vi "Autonomous_v204.vi"() -> ()   [LabVIEW 2017]
doc: "This VI starts when autonomous period begins, and will automatically be terminated when it ends. You can carry out timed or sensor driven operations directly to I/O or to subsystems without needing to return to the caller."
uses:
  <vilib>/Rock Robotics/Network Tables/NT Read String.vi
panel:
  out "RightArmMotorCmd 2":dbl(graph)
  out "Lift Min Limit  2":bool
  out "Lift Max Limit 2":bool
  out "LiftMotorCmd 2":dbl(graph)
  out "Left Arm Max Limit 2":bool
  out "Right Arm Max Limit 2":bool
  out "Right Arm Min Limit 2":bool
  out "Left Arm Min Limit 2":bool
  out "LeftArmMotorCmd 2":dbl(graph)
  out "Arm Lift Min Limit  2":bool
  out "Arm Lift Max Limit  2":bool
  out "ArmLiftMotorCmd 2":dbl(graph)
  out "Waveform Chart 6":dbl(graph)
  out "Waveform Chart 15":dbl(graph)
  out "Waveform Chart 10":dbl(graph)
  out "millisecond timer value 3":u32
  out "String 2":string
  out "Waveform Chart 45":i32(graph)
  out "Waveform Chart 44":i32(graph)
  out "Waveform Chart 43":i32(graph)
  out "Waveform Chart 42":i32(graph)
  out "Waveform Chart 14":i32(graph)
  out "Waveform Chart 12":i32(graph)
  out "Waveform Chart 41":i32(graph)
  out "Waveform Chart 40":i32(graph)
  out "Waveform Chart 39":i32(graph)
  out "Waveform Chart 38":i32(graph)
  out "Waveform Chart 37":i32(graph)
  out "Waveform Chart 36":i32(graph)
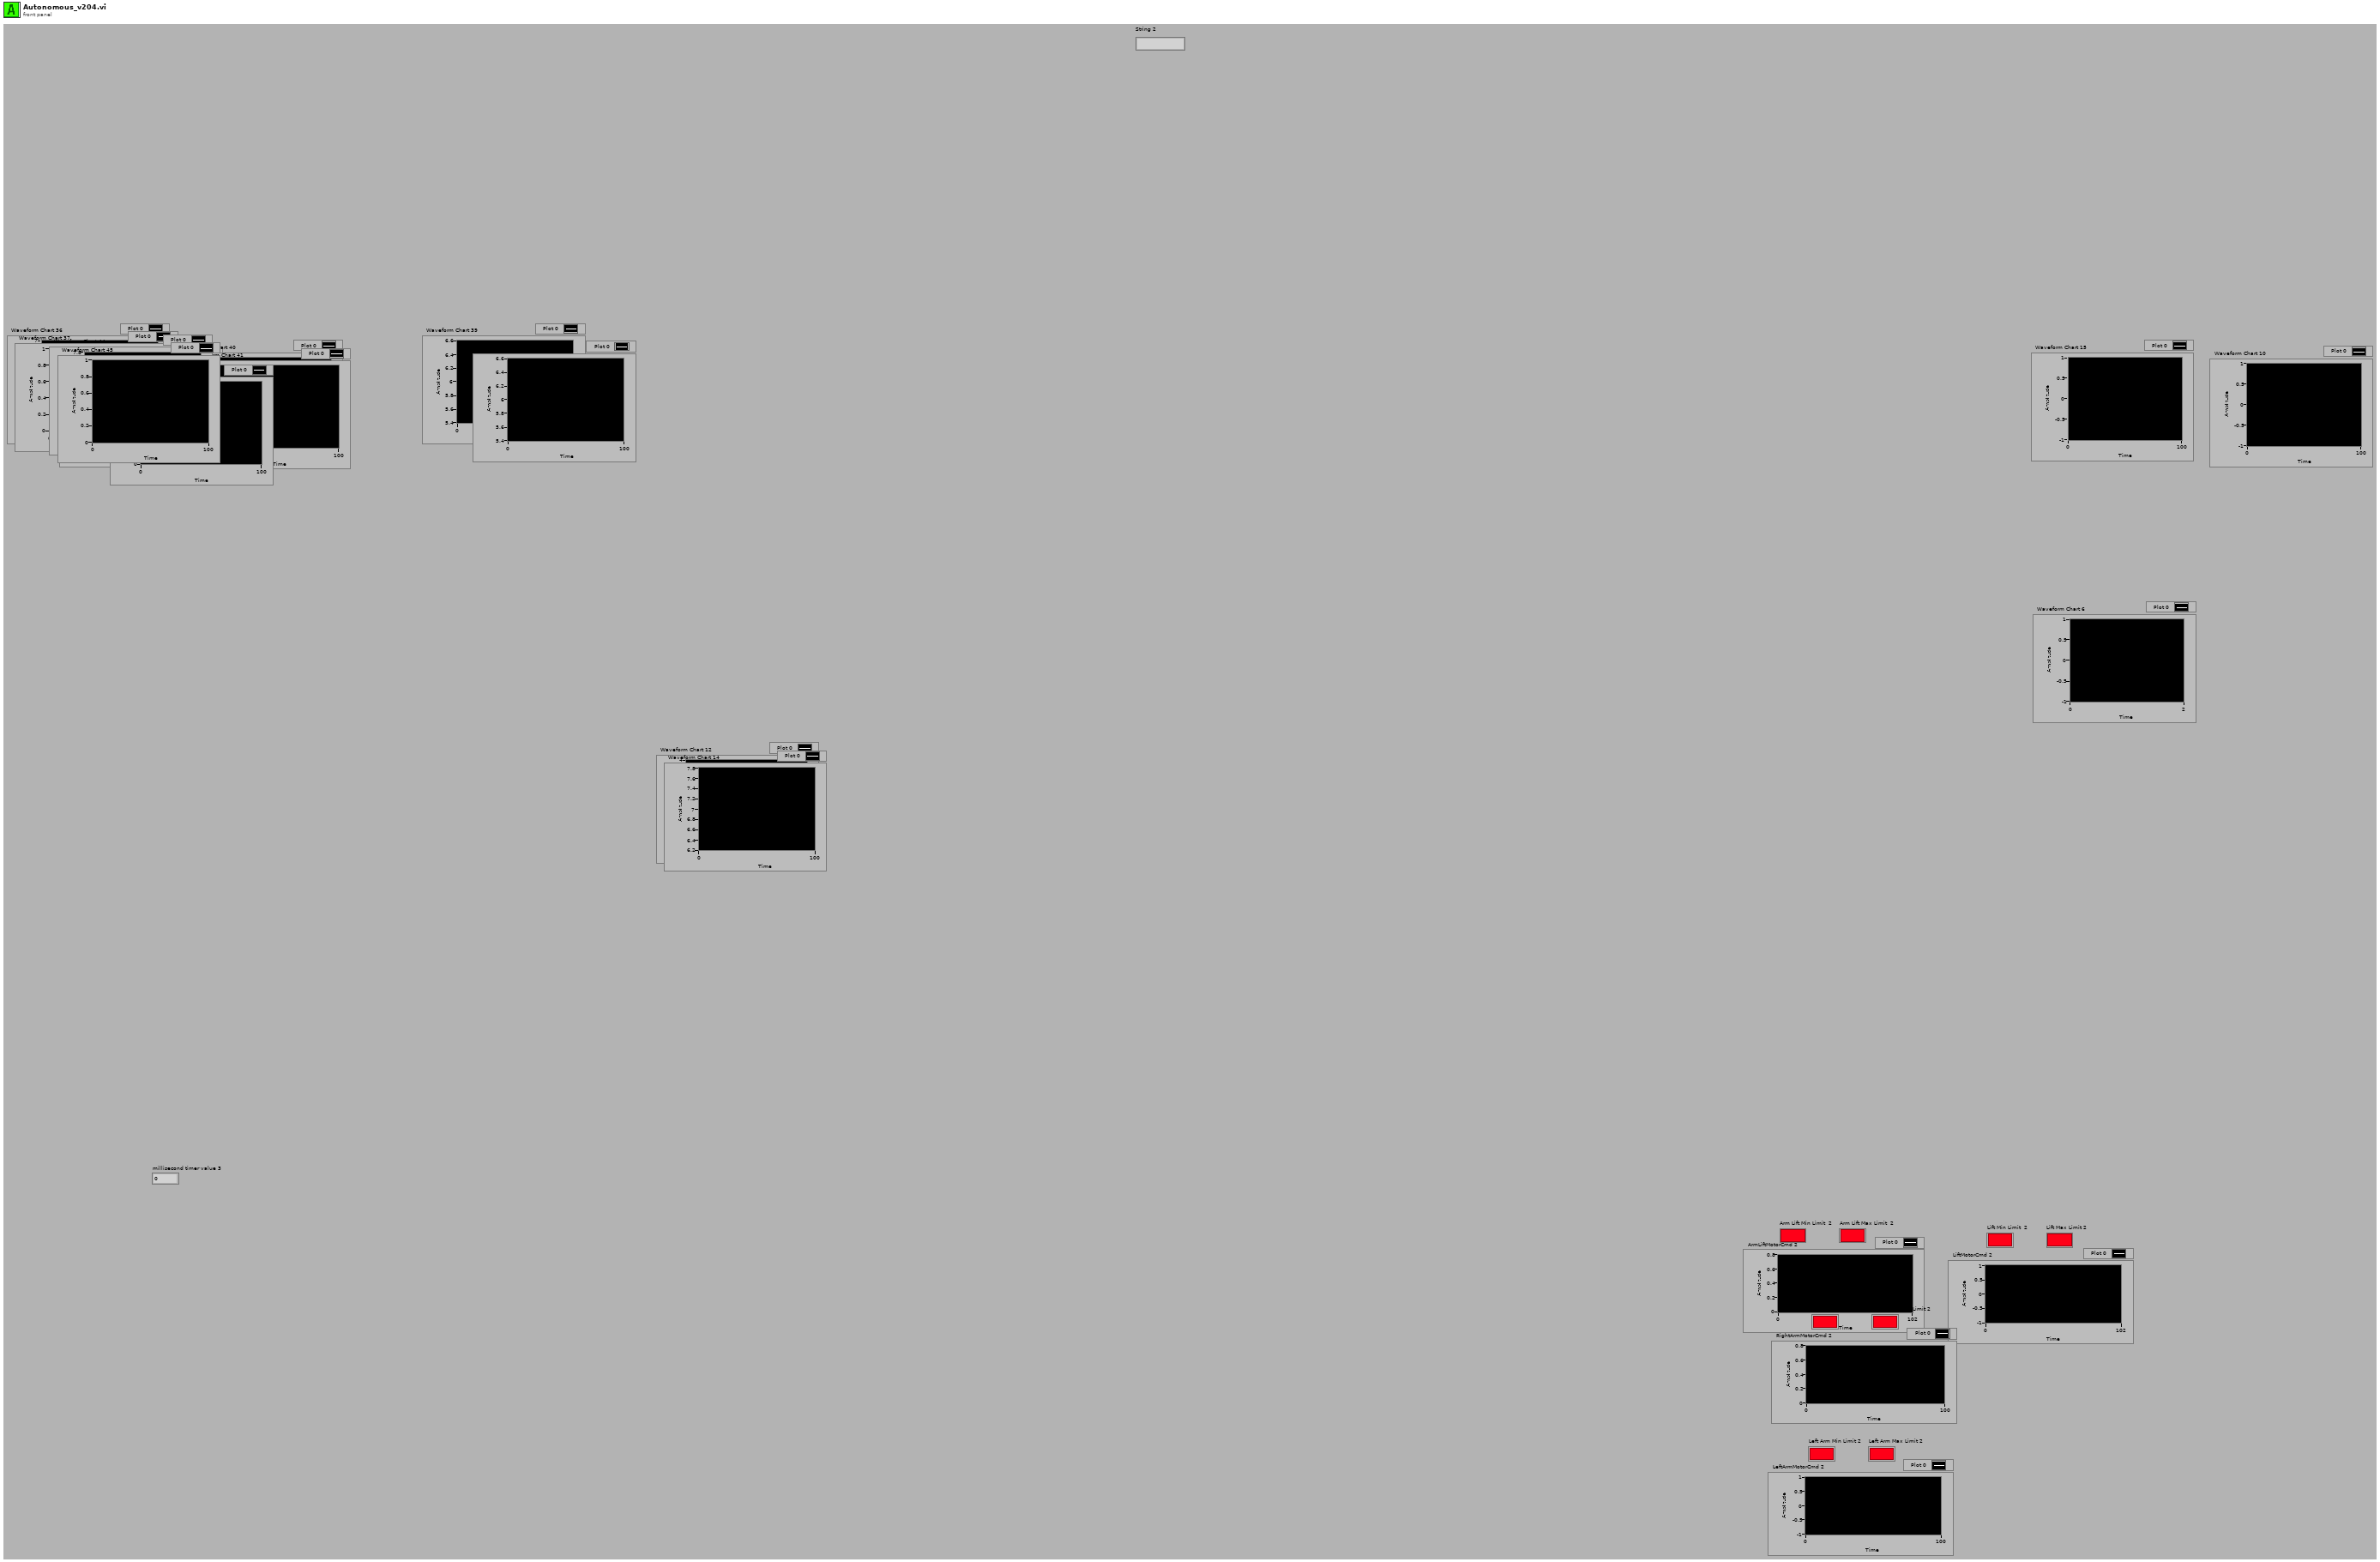
[diagram p1: front panel]
types:
  T1 = cluster{"X_axis":dbl, "Y_axis":dbl, "RotationTarget":dbl, "ArmLift":dbl, "Hands":dbl, "Lift":dbl, "Arms":dbl}
  T2 = enum16{"initialize", "read", "write", "write all"}
  T3 = typedef "DioDisplayALB.ctl" = cluster{"DIO 0-LiftMinLimitSwitch":bool, "DIO 1-LiftMaxLimitSwitch":bool, "DIO 2-LiftArmMinLimitSwitch":bool, "DIO 3-LiftArmMaxLimitSwitch":bool, "DIO 4-RightArmMaxLimitSwitch":bool, "DIO 5-RightArmMinLimitSwitch":bool, "DIO 6-LeftArmMaxLimitSwitch":bool, "DIO 7-LeftArmMinLimitSwitch":bool, "DIO 8":bool, "DIO 9":bool}
  T4 = typedef "WPI_MotorControlDeviceRef.ctl" = cluster{"DeviceStatus":errorcluster, "Type":T5, "PWM":cluster{"PWM Channel":T6, "DeadBand":T7}, "CAN":cluster{"Device Number":u8, "SetOutput VI Ref":variant, "GetOutput VI Ref":variant, "Enable VI Ref":variant, "Disable VI Ref":variant, "Data":variant}, "Invert":bool, "DIO PWM":cluster{"PWM \"Enable\" Channel":T6, "DIOChannel":T8, "PWM Rate":dbl}}
  T5 = typedef "WPI_MotorControlType.ctl" = enum16{"PWM", "CAN", "DIO PWM"}
  T6 = typedef "FPGA_DIOPWMChannel.ctl" = enum8{"PWM 0", "PWM 1", "PWM 2", "PWM 3", "PWM 4", "PWM 5", "PWM 6", "PWM 7", "PWM 8", "PWM 9", "PWM MXP 0", "PWM MXP 1", "PWM MXP 2", "PWM MXP 3", "PWM MXP 4", "PWM MXP 5", "PWM MXP 6", "PWM MXP 7", "PWM MXP 8", "PWM MXP 9", "Invalid"}
  T7 = typedef "WPI_PWMDeadband.ctl" = cluster{"Name":string, "maxPositivePwm":i32, "minPositivePwm":i32, "centerPwm":i32, "maxNegativePwm":i32, "minNegativePwm":i32, "angularRange":u16}
  T8 = typedef "FPGA_DIOChannel.ctl" = enum8{"DIO 0", "DIO 1", "DIO 2", "DIO 3", "DIO 4", "DIO 5", "DIO 6", "DIO 7", "DIO 8", "DIO 9", "DIO MXP 0", "DIO MXP 1", "DIO MXP 2", "DIO MXP 3", "DIO MXP 4", "DIO MXP 5", "DIO MXP 6", "DIO MXP 7", "DIO MXP 8", "DIO MXP 9", "DIO MXP 10", "DIO MXP 11", "DIO MXP 12", "DIO MXP 13", "DIO MXP 14", "DIO MXP 15", "SPI Port CS1", "SPI Port CS2", "SPI Port CS3", "SPI Port MISO", "SPI Port MOSI", "Invalid"}
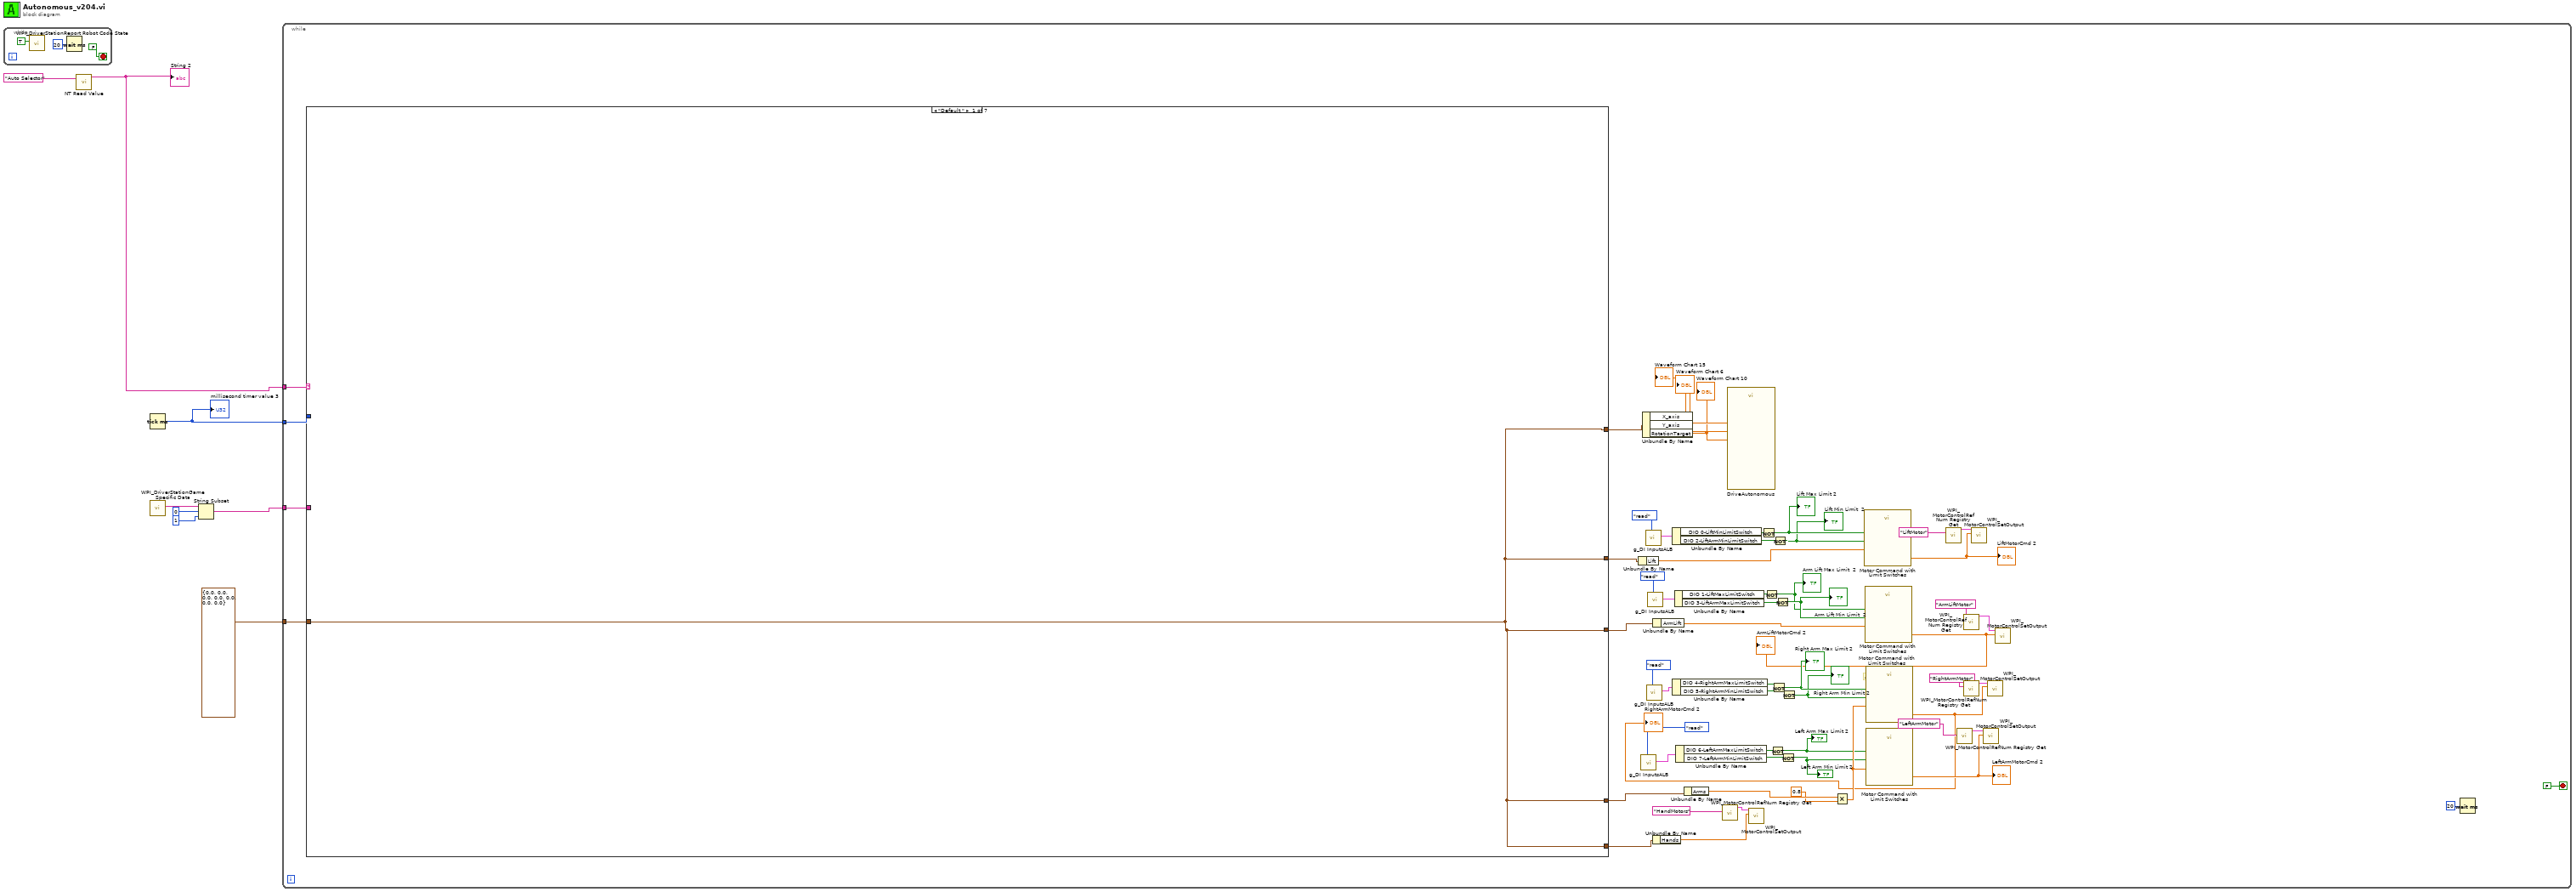
[diagram p0: block diagram]
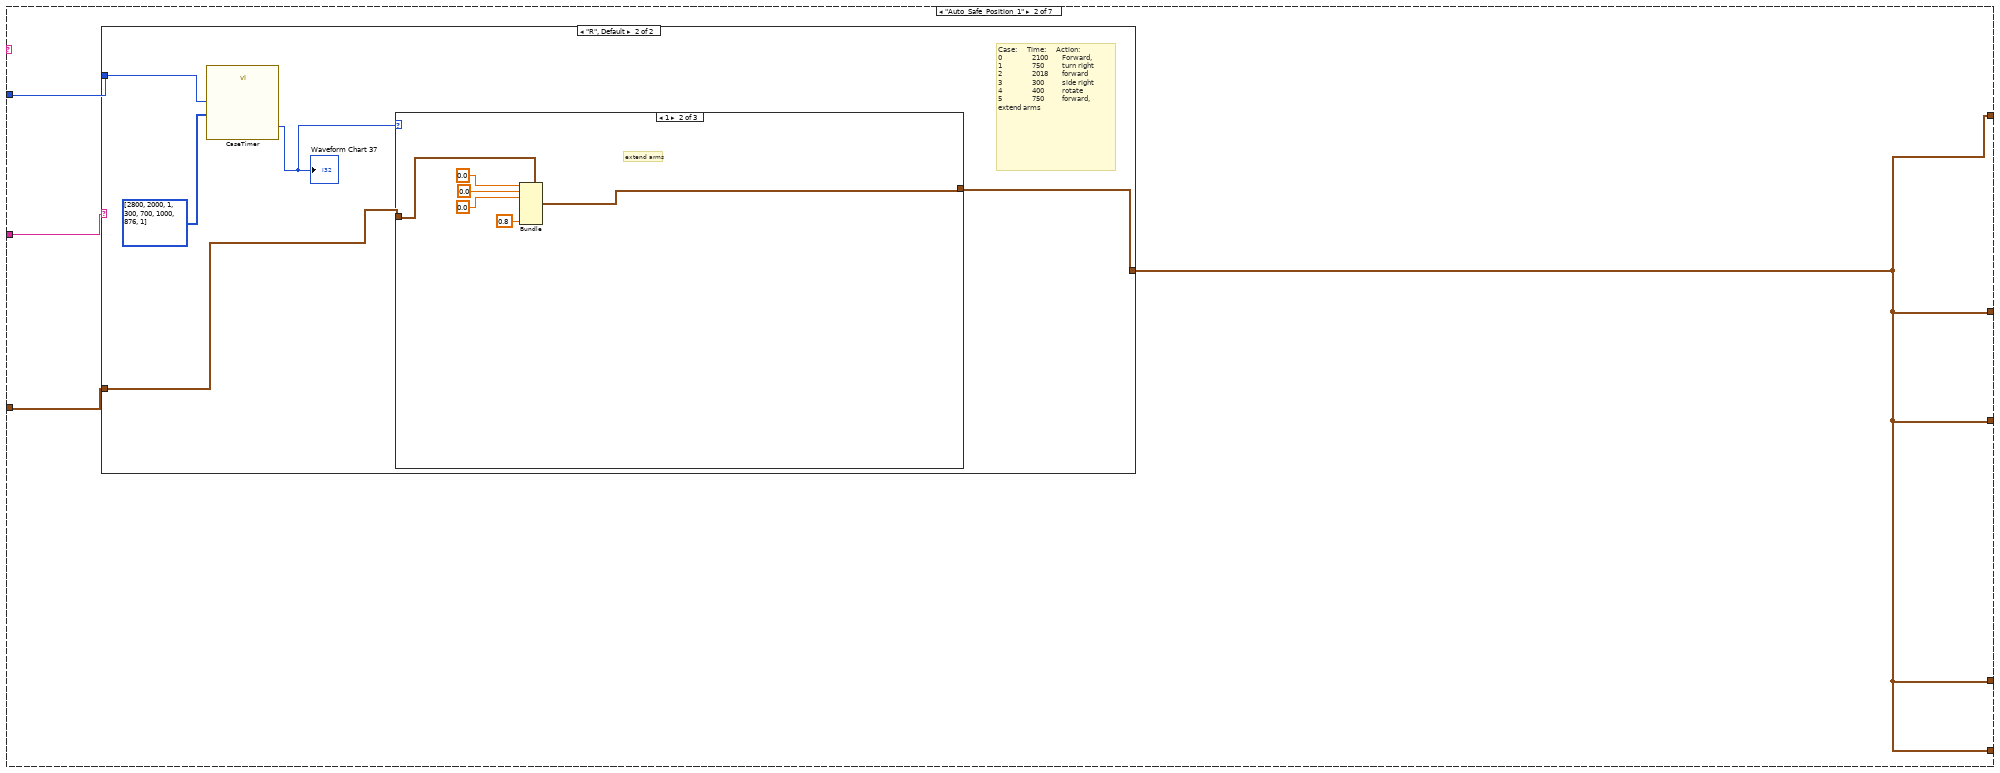
[diagram p2: hidden frame]
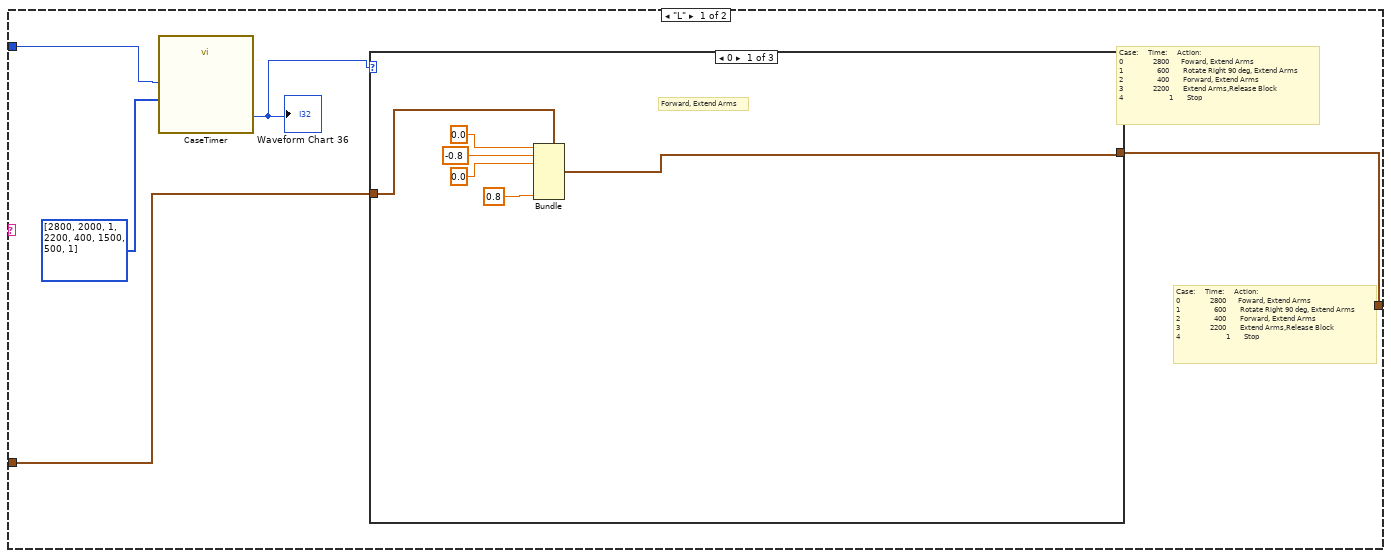
[diagram p3: hidden frame]
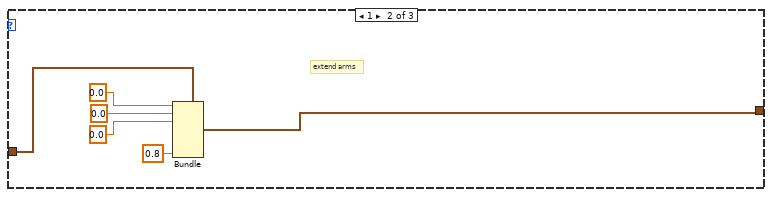
[diagram p4: hidden frame]
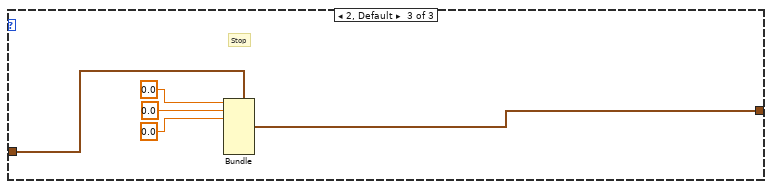
[diagram p5: hidden frame]
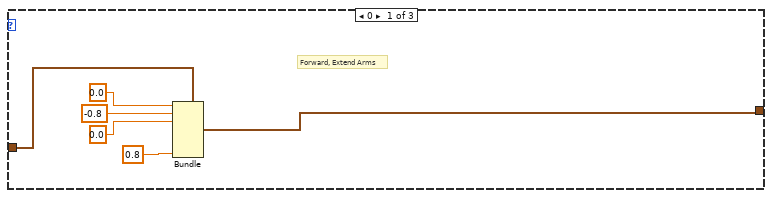
[diagram p6: hidden frame]
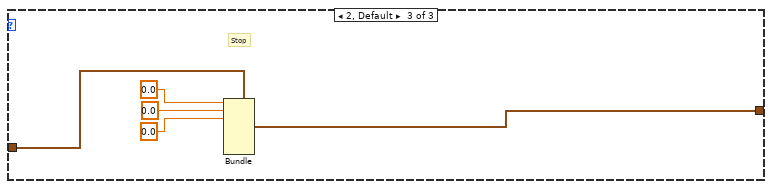
[diagram p7: hidden frame]
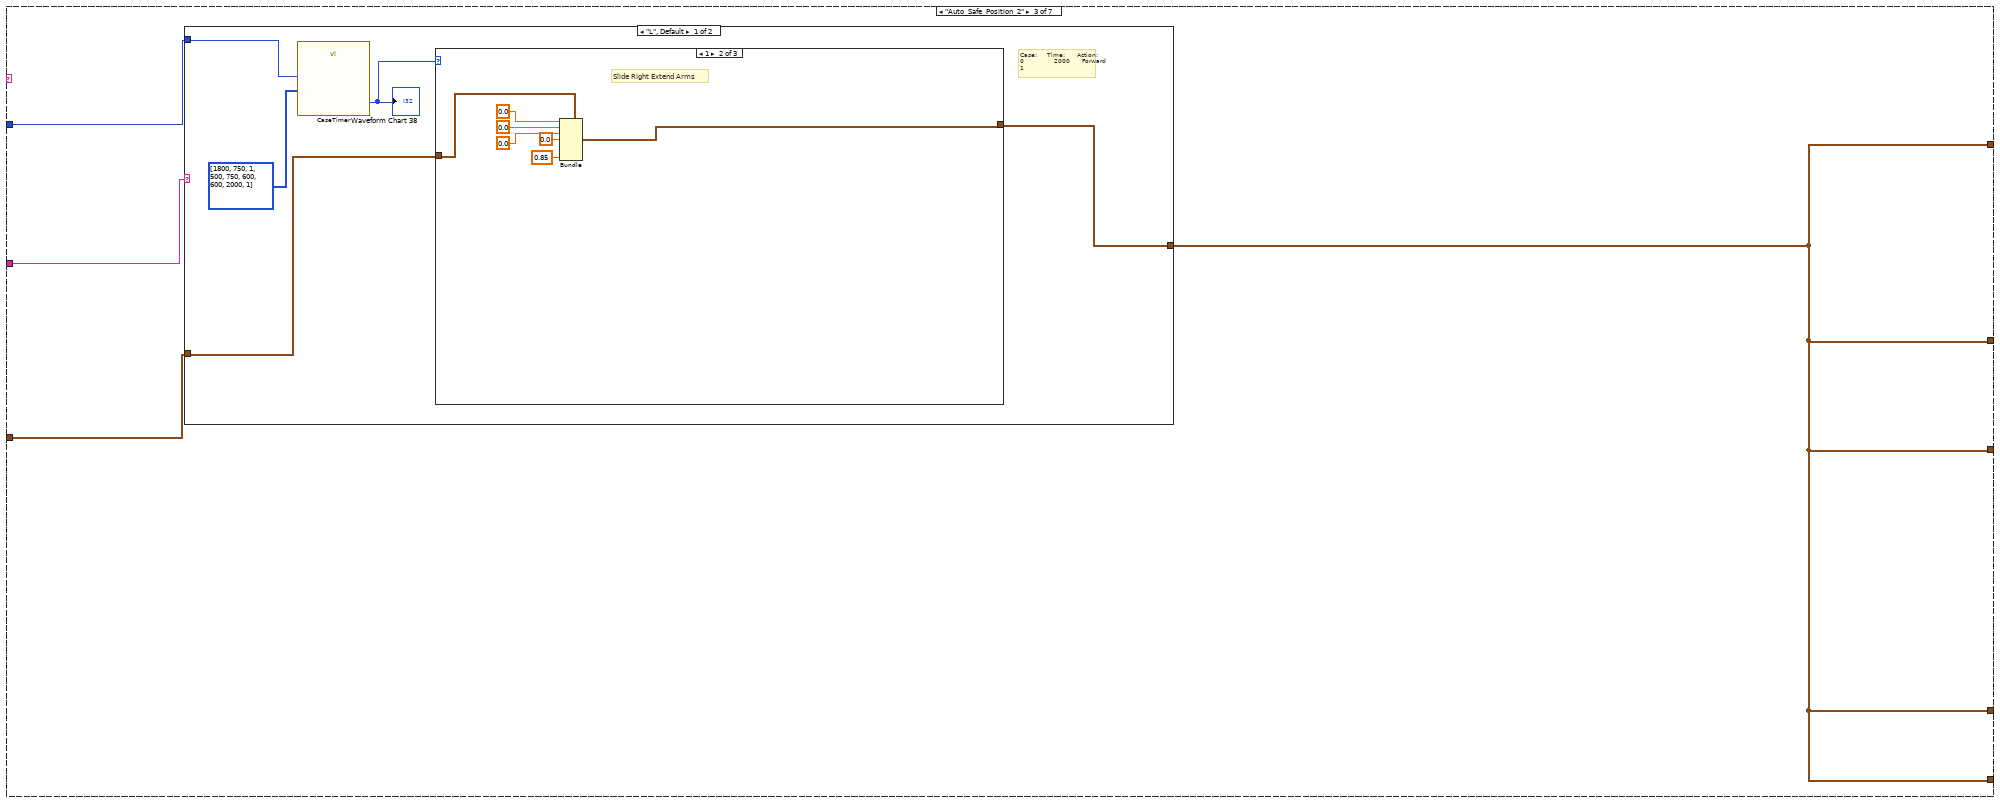
[diagram p8: hidden frame]
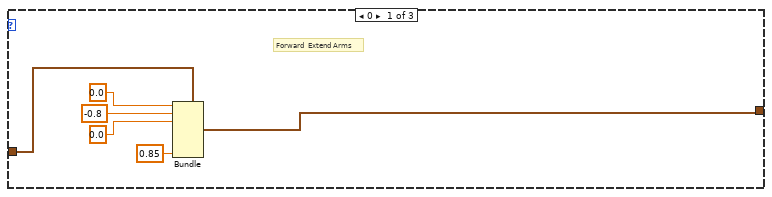
[diagram p9: hidden frame]
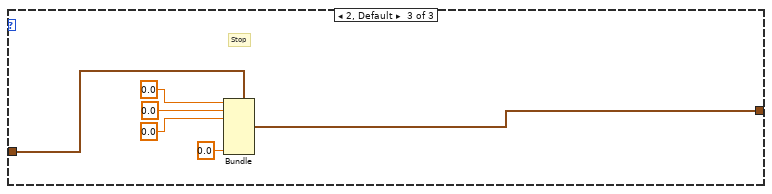
[diagram p10: hidden frame]
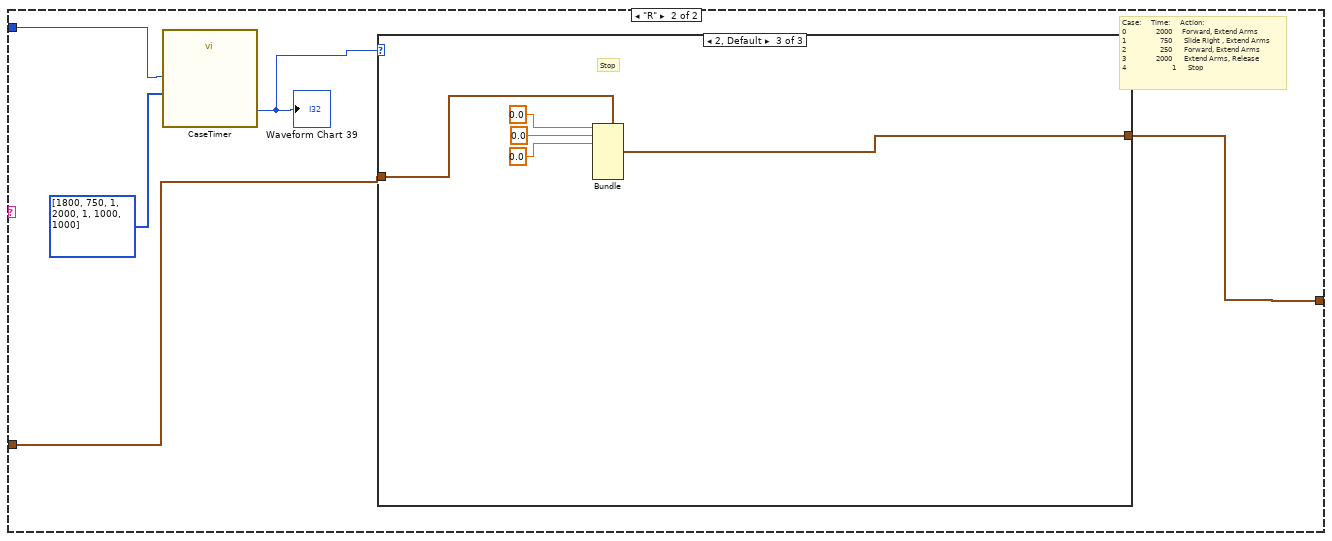
[diagram p11: hidden frame]
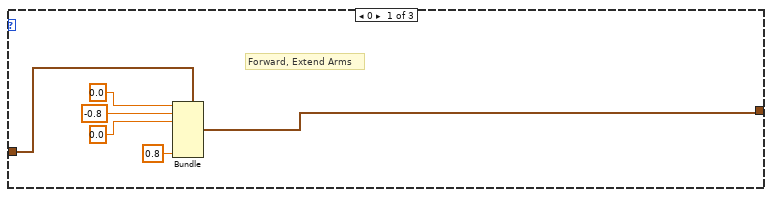
[diagram p12: hidden frame]
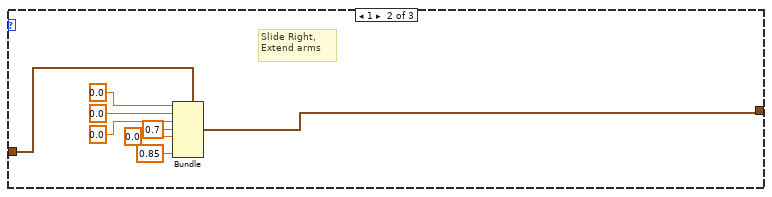
[diagram p13: hidden frame]
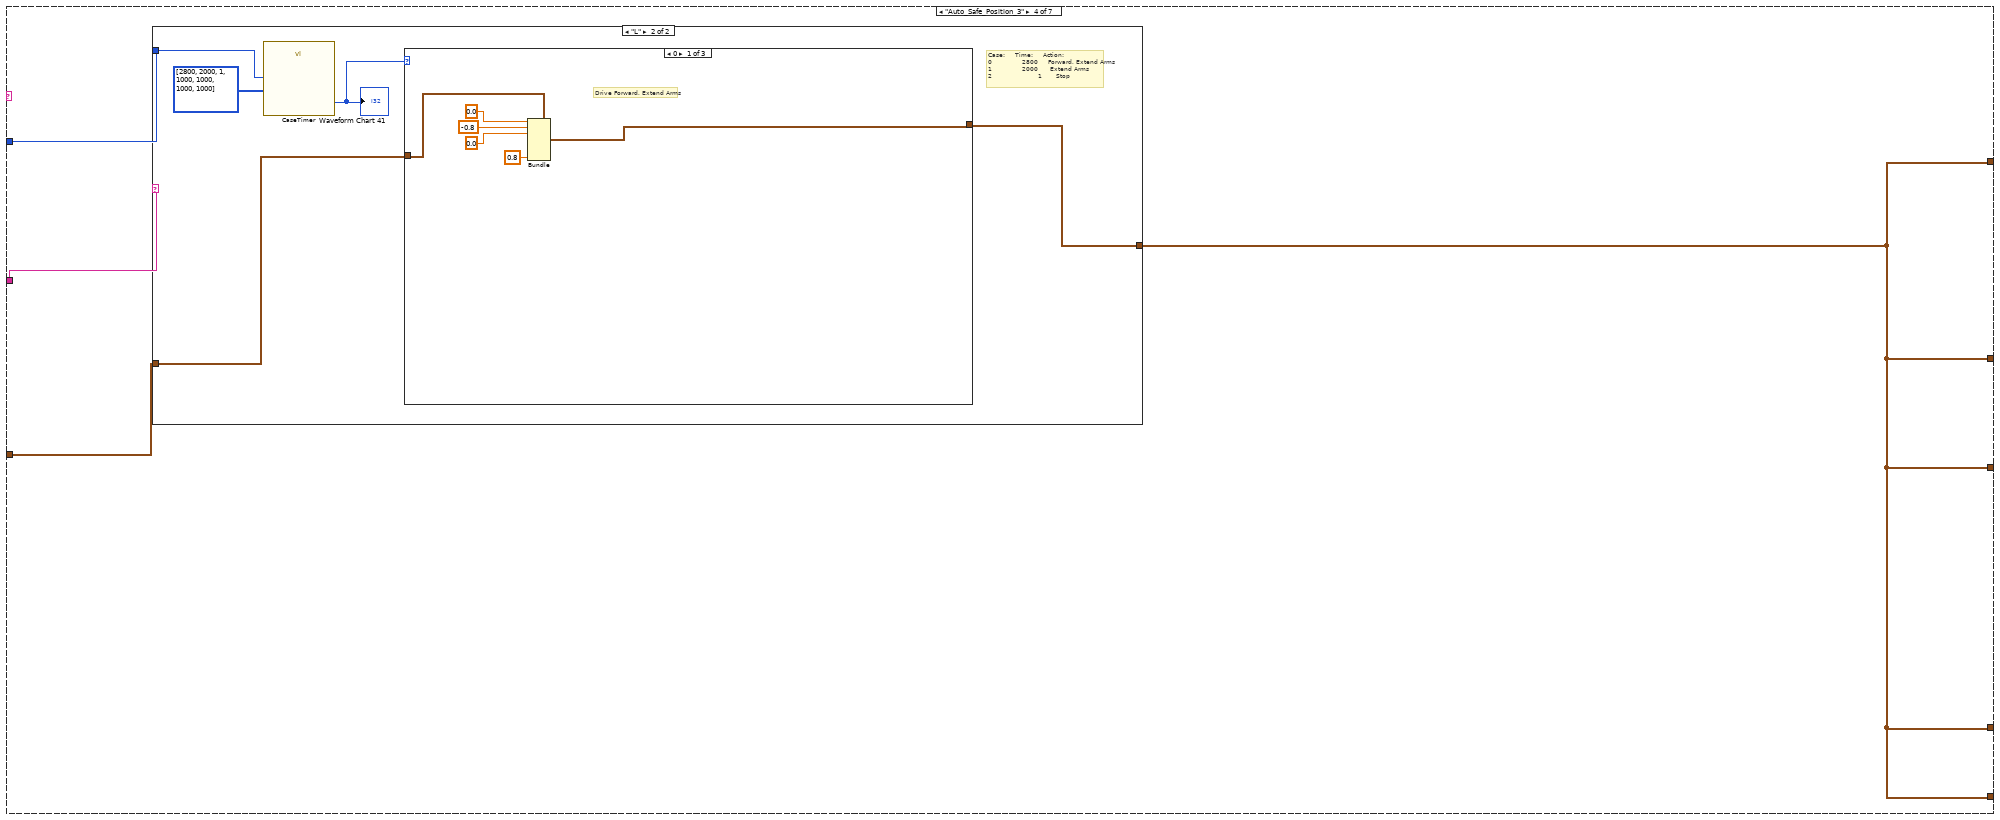
[diagram p14: hidden frame]
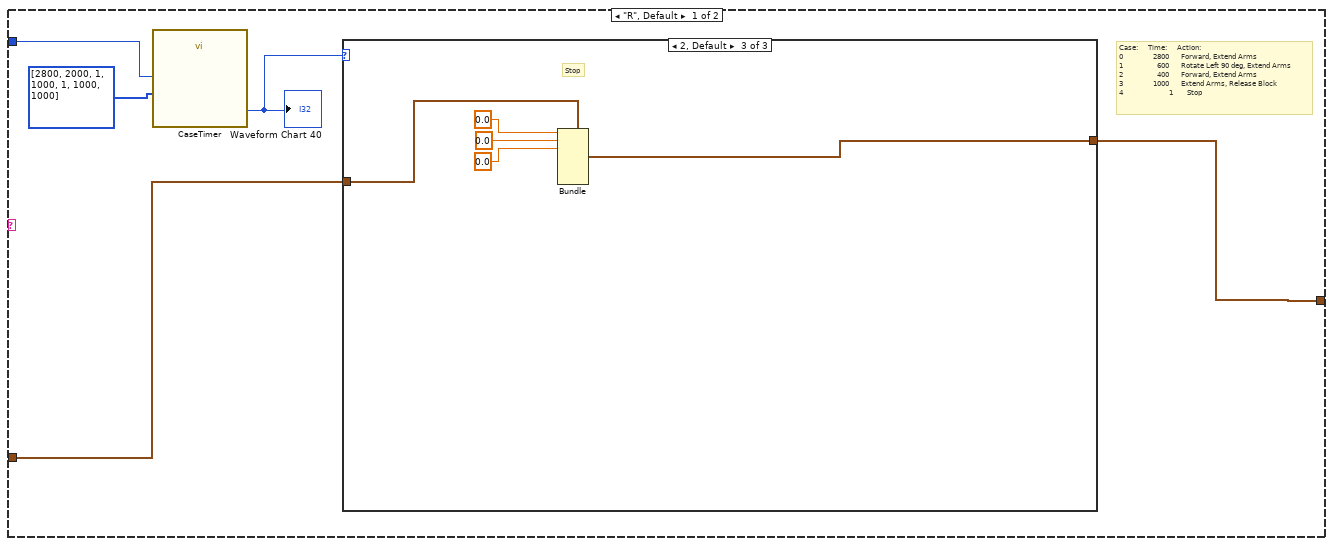
[diagram p15: hidden frame]
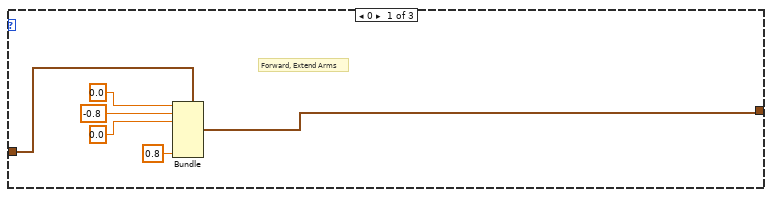
[diagram p16: hidden frame]
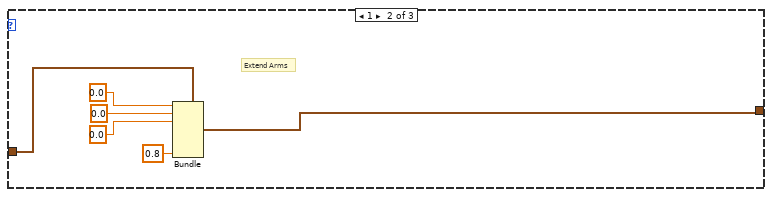
[diagram p17: hidden frame]
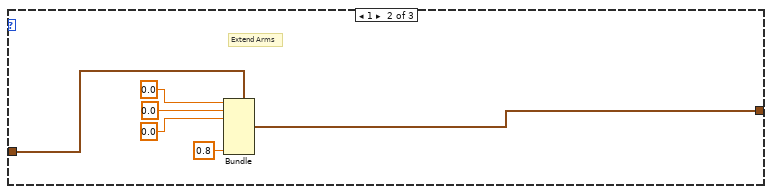
[diagram p18: hidden frame]
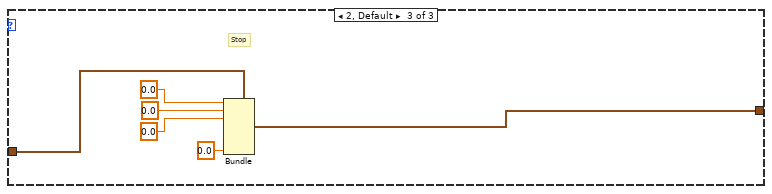
[diagram p19: hidden frame]
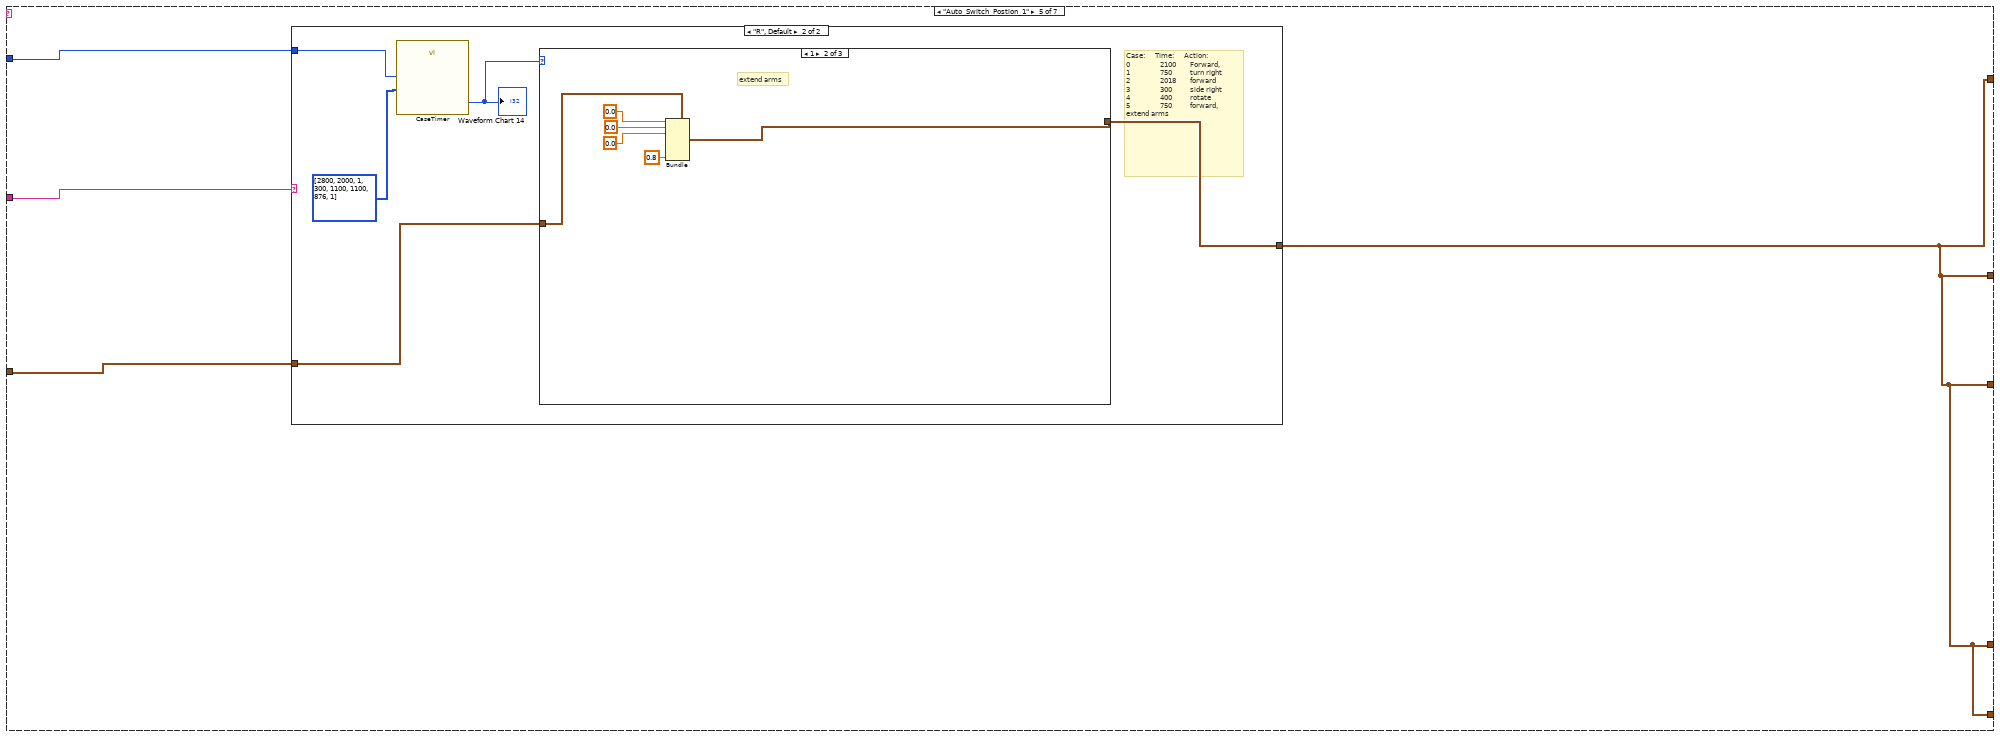
[diagram p20: hidden frame]
diagram:
  n1 = while {
    stop <- FALSE stop-if-true
    n2 = call <vilib>:"WPI_DriverStationReport Robot Code State.vi"("Autonomous"=TRUE) -> ()  [unwired: 10 in, 1 out]
    n3 = Wait (ms)(milliseconds to wait=u32 20) -> ()  [unwired: 1 out]
  }
  n4 = call-poly <vilib>:"NT Read Value.vi"("Name"="Auto Selector") -> ("String"=w1:string)  [unwired: 9 in, 1 out]
  "String 2" <- w1
  n5 = call <vilib>:"WPI_DriverStationGame Specific Data.vi"() -> ("Game Specific Data"=w7:string)  [unwired: 11 in]
  n6 = Tick Count (ms)() -> (millisecond timer value=w2:u32)
  "millisecond timer value 3" <- w2
  n7 = String Subset(string=w7, offset (0)=0, length (rest)=1 ("length (rest)")) -> (substring=w3:string)
  n8 = while {
    tunnel: T1 {"X_axis"=0.0, "Y_axis"=0.0, "RotationTarget"=0.0, "ArmLift"=0.0, "Hands"=0.0, "Lift"=0.0, "Arms"=0.0} ("Cluster") -> [w68]
    tunnel: w3 -> [w67]
    tunnel: w2 -> [w66]
    tunnel: w1 -> [w65]
    stop <- FALSE stop-if-true
    # "Arms"
    n9 = case shown="\"Default \"" w65 {
      tunnel: w66 -> [_ w73 w119 w174 w222 w302 w359]
      tunnel: w68 -> [w70 w72 w121 w172 w221 w300 w361]
      tunnel: w67 -> [_ w74 w122 w173 w223 w301 w362]
      tunnel: [w70 w71 w120 w171 w220 w299 w360] -> w15
      tunnel: [w70 w71 w120 w171 w220 w299 w360] -> w17
      tunnel: [w70 w71 w120 w171 w220 w299 w360] -> w16
      tunnel: [w70 w71 w120 w171 w220 w299 w360] -> w14
      tunnel: [w70 w71 w120 w171 w220 w299 w360] -> w18
      frame "Default " {
      }
      frame "Auto_Safe_Position_1" {
        n10 = case shown="\"R\", Default" w74 {
          tunnel: w72 -> [w77 w99]
          tunnel: [w75 w97] -> w71
          tunnel: w73 -> [w79 w101]
          frame "L" {
            # "Case:     Time:     Action:\n0               2800      Foward, Extend Arms\n1                 600       Rotate Right 90 deg, Extend Arms\n2                 400       Forward, Extend Arms\n3               2200       Extend Arms,Release Block\n4                       1       Stop"
            # "Case:     Time:     Action:\n0               2800      Foward, Extend Arms\n1                 600       Rotate Right 90 deg, Extend Arms\n2                 400       Forward, Extend Arms\n3               2200       Extend Arms,Release Block\n4                       1       Stop"
            n11 = call "CaseTimer.vi"("CaseTime"=u32[] [2800, 2000, 1, 2200, 400, 1500, 500, 1] ("y"), "ElapsedTime"=w79) -> ("CaseNumber"=w76:i32)  [unwired: 9 in]
            "Waveform Chart 36" <- w76
            n12 = case shown="0" w76 {
              tunnel: [w82 w88 w93] -> w75
              tunnel: w77 -> [w80 w86 w92]
              frame 0 {
                # "Forward, Extend Arms"
                n13 = Bundle(cluster=w80, "X_axis"=0.0, "Y_axis"=-0.8, "RotationTarget"=0.0, "Arms"=0.8) -> (w82:T1)  [unwired: 3 in]
              }
              frame 1 {
                # "extend arms"
                n14 = Bundle(cluster=w86, "X_axis"=0.0, "Y_axis"=0.0, "RotationTarget"=0.0, "Arms"=0.8) -> (w88:T1)  [unwired: 3 in]
              }
              frame 2, Default {
                # "Stop"
                n15 = Bundle(cluster=w92, "X_axis"=0.0, "Y_axis"=0.0, "RotationTarget"=0.0) -> (w93:T1)  [unwired: 4 in]
              }
            }
          }
          frame "R", Default {
            # "Case:     Time:     Action:\n0               2100       Forward, \n1               750         turn right\n2               2018       forward\n3               300         side right\n4               400         rotate\n5               750         forward, extend arms"
            n16 = call "CaseTimer.vi"("CaseTime"=u32[] [2800, 2000, 1, 300, 700, 1000, 876, 1] ("y"), "ElapsedTime"=w101) -> ("CaseNumber"=w98:i32)  [unwired: 9 in]
            "Waveform Chart 37" <- w98
            n17 = case shown="1" w98 {
              tunnel: [w104 w110 w115] -> w97
              tunnel: w99 -> [w102 w108 w114]
              frame 0 {
                # "Forward, Extend Arms"
                n18 = Bundle(cluster=w102, "X_axis"=0.0, "Y_axis"=-0.8, "RotationTarget"=0.0, "Arms"=0.8) -> (w104:T1)  [unwired: 3 in]
              }
              frame 1 {
                # "extend arms"
                n19 = Bundle(cluster=w108, "X_axis"=0.0, "Y_axis"=0.0, "RotationTarget"=0.0, "Arms"=0.8) -> (w110:T1)  [unwired: 3 in]
              }
              frame 2, Default {
                # "Stop"
                n20 = Bundle(cluster=w114, "X_axis"=0.0, "Y_axis"=0.0, "RotationTarget"=0.0) -> (w115:T1)  [unwired: 4 in]
              }
            }
          }
        }
      }
      frame "Auto_Safe_Position_2" {
        n21 = case shown="\"L\", Default" w122 {
          tunnel: w121 -> [w127 w149]
          tunnel: [w126 w147] -> w120
          tunnel: w119 -> [w124 w151]
          frame "L", Default {
            # "Case:     Time:      Action:\n0               2000      Forward\n1"
            n22 = call "CaseTimer.vi"("CaseTime"=u32[] [1800, 750, 1, 500, 750, 600, 600, 2000, 1] ("y"), "ElapsedTime"=w124) -> ("CaseNumber"=w125:i32)  [unwired: 9 in]
            "Waveform Chart 38" <- w125
            n23 = case shown="1" w125 {
              tunnel: w127 -> [w130 w137 w146]
              tunnel: [w129 w136 w142] -> w126
              frame 0 {
                # "Forward  Extend Arms"
                n24 = Bundle(cluster=w130, "X_axis"=0.0, "Y_axis"=-0.8, "RotationTarget"=0.0, "Arms"=0.85) -> (w129:T1)  [unwired: 3 in]
              }
              frame 1 {
                # "Slide RIght Extend Arms"
                n25 = Bundle(cluster=w137, "X_axis"=0.0, "Y_axis"=0.0, "RotationTarget"=0.0, "ArmLift"=0.0, "Arms"=0.85) -> (w136:T1)  [unwired: 2 in]
              }
              frame 2, Default {
                # "Stop"
                n26 = Bundle(cluster=w146, "X_axis"=0.0, "Y_axis"=0.0, "RotationTarget"=0.0, "Arms"=0.0) -> (w142:T1)  [unwired: 3 in]
              }
            }
          }
          frame "R" {
            # "Case:     Time:     Action:\n0               2000     Forward, Extend Arms\n1                 750      Slide Right , Extend Arms\n2                 250      Forward, Extend Arms\n3               2000      Extend Arms, Release\n4                       1      Stop"
            n27 = call "CaseTimer.vi"("CaseTime"=u32[] [1800, 750, 1, 2000, 1, 1000, 1000] ("y"), "ElapsedTime"=w151) -> ("CaseNumber"=w148:i32)  [unwired: 9 in]
            "Waveform Chart 39" <- w148
            n28 = case shown="2, Default" w148 {
              tunnel: w149 -> [w154 w162 w170]
              tunnel: [w153 w161 w166] -> w147
              frame 0 {
                # "Forward, Extend Arms"
                n29 = Bundle(cluster=w154, "X_axis"=0.0, "Y_axis"=-0.8, "RotationTarget"=0.0, "Arms"=0.8) -> (w153:T1)  [unwired: 3 in]
              }
              frame 1 {
                # "Slide Right, Extend arms"
                n30 = Bundle(cluster=w162, "X_axis"=0.0, "Y_axis"=0.0, "RotationTarget"=0.0, "ArmLift"=0.7, "Hands"=0.0, "Arms"=0.85) -> (w161:T1)  [unwired: 1 in]
              }
              frame 2, Default {
                # "Stop"
                n31 = Bundle(cluster=w170, "X_axis"=0.0, "Y_axis"=0.0, "RotationTarget"=0.0) -> (w166:T1)  [unwired: 4 in]
              }
            }
          }
        }
      }
      frame "Auto_Safe_Position_3" {
        n32 = case shown="\"L\"" w173 {
          tunnel: w172 -> [w179 w201]
          tunnel: [w178 w200] -> w171
          tunnel: w174 -> [w176 w198]
          frame "R", Default {
            # "Case:     Time:     Action:\n0               2800      Forward, Extend Arms\n1                 600      Rotate Left 90 deg, Extend Arms\n2                 400      Forward, Extend Arms\n3               1000      Extend Arms, Release Block\n4                       1       Stop"
            n33 = call "CaseTimer.vi"("CaseTime"=u32[] [2800, 2000, 1, 1000, 1, 1000, 1000] ("y"), "ElapsedTime"=w176) -> ("CaseNumber"=w177:i32)  [unwired: 9 in]
            "Waveform Chart 40" <- w177
            n34 = case shown="2, Default" w177 {
              tunnel: w179 -> [w182 w188 w196]
              tunnel: [w181 w187 w192] -> w178
              frame 0 {
                # "Forward, Extend Arms"
                n35 = Bundle(cluster=w182, "X_axis"=0.0, "Y_axis"=-0.8, "RotationTarget"=0.0, "Arms"=0.8) -> (w181:T1)  [unwired: 3 in]
              }
              frame 1 {
                # "Extend Arms"
                n36 = Bundle(cluster=w188, "X_axis"=0.0, "Y_axis"=0.0, "RotationTarget"=0.0, "Arms"=0.8) -> (w187:T1)  [unwired: 3 in]
              }
              frame 2, Default {
                # "Stop"
                n37 = Bundle(cluster=w196, "X_axis"=0.0, "Y_axis"=0.0, "RotationTarget"=0.0) -> (w192:T1)  [unwired: 4 in]
              }
            }
          }
          frame "L" {
            # "Case:     Time:     Action:\n0               2800     Forward, Extend Arms\n1               2000      Extend Arms\n2                       1       Stop"
            n38 = call "CaseTimer.vi"("CaseTime"=u32[] [2800, 2000, 1, 1000, 1000, 1000, 1000] ("y"), "ElapsedTime"=w198) -> ("CaseNumber"=w199:i32)  [unwired: 9 in]
            "Waveform Chart 41" <- w199
            n39 = case shown="0" w199 {
              tunnel: w201 -> [w204 w213 w219]
              tunnel: [w203 w209 w215] -> w200
              frame 0 {
                # "Drive Forward, Extend Arms"
                n40 = Bundle(cluster=w204, "X_axis"=0.0, "Y_axis"=-0.8, "RotationTarget"=0.0, "Arms"=0.8) -> (w203:T1)  [unwired: 3 in]
              }
              frame 1 {
                # "Extend Arms"
                n41 = Bundle(cluster=w213, "X_axis"=0.0, "Y_axis"=0.0, "RotationTarget"=0.0, "Arms"=0.8) -> (w209:T1)  [unwired: 3 in]
              }
              frame 2, Default {
                # "Stop"
                n42 = Bundle(cluster=w219, "X_axis"=0.0, "Y_axis"=0.0, "RotationTarget"=0.0, "Arms"=0.0) -> (w215:T1)  [unwired: 3 in]
              }
            }
          }
        }
      }
      frame "Auto_Switch_Postion_1" {
        n43 = case shown="\"R\", Default" w223 {
          tunnel: w221 -> [w228 w280]
          tunnel: [w227 w279] -> w220
          tunnel: w222 -> [w226 w277]
          frame "L" {
            # "Case:     Time:     Action:\n0               2800      Foward, Extend Arms\n1                 600       Rotate Right 90 deg, Extend Arms\n2                 400       Forward, Extend Arms\n3               2200       Extend Arms,Release Block\n4                       1       Stop"
            n44 = call "CaseTimer.vi"("CaseTime"=u32[] [2800, 660, 400, 2200, 400, 1500, 500, 1] ("y"), "ElapsedTime"=w226) -> ("CaseNumber"=w225:i32)  [unwired: 9 in]
            "Waveform Chart 12" <- w225
            n45 = case shown="0" w225 {
              tunnel: w228 -> [w231 w237 w243 w253 w255 w261 w267 w275]
              tunnel: [w230 w236 w242 w249 w254 w260 w266 w271] -> w227
              frame 0 {
                # "Forward, Extend Arms"
                n46 = Bundle(cluster=w231, "X_axis"=0.0, "Y_axis"=-0.8, "RotationTarget"=0.0, "Arms"=0.8) -> (w230:T1)  [unwired: 3 in]
              }
              frame 1 {
                # "Rotate Right 90 deg"
                n47 = Bundle(cluster=w237, "X_axis"=1.0, "Y_axis"=0.0, "RotationTarget"=0.0, "Arms"=0.8) -> (w236:T1)  [unwired: 3 in]
              }
              frame 2 {
                n48 = Bundle(cluster=w243, "X_axis"=0.0, "Y_axis"=-1.0, "RotationTarget"=0.0, "Arms"=0.8) -> (w242:T1)  [unwired: 3 in]
              }
              frame 3 {
                # "Extend Arms, Release Block"
                n49 = Bundle(cluster=w253, "X_axis"=0.0, "Y_axis"=0.0, "RotationTarget"=0.0, "Hands"=-1.0, "Arms"=0.8) -> (w249:T1)  [unwired: 2 in]
              }
              frame 4 {
                # "backup"
                n50 = Bundle(cluster=w255, "X_axis"=0.0, "Y_axis"=1.0, "RotationTarget"=0.0, "Arms"=0.0) -> (w254:T1)  [unwired: 3 in]
              }
              frame 5 {
                # "slide left"
                n51 = Bundle(cluster=w261, "X_axis"=0.0, "Y_axis"=0.0, "RotationTarget"=-0.7, "Arms"=0.0) -> (w260:T1)  [unwired: 3 in]
              }
              frame 6 {
                # "Forward"
                n52 = Bundle(cluster=w267, "X_axis"=0.0, "Y_axis"=-1.0, "RotationTarget"=0.0) -> (w266:T1)  [unwired: 4 in]
              }
              frame 7, Default {
                # "Stop"
                n53 = Bundle(cluster=w275, "X_axis"=0.0, "Y_axis"=0.0, "RotationTarget"=0.0) -> (w271:T1)  [unwired: 4 in]
              }
            }
          }
          frame "R", Default {
            # "Case:     Time:     Action:\n0               2100       Forward, \n1               750         turn right\n2               2018       forward\n3               300         side right\n4               400         rotate\n5               750         forward, extend arms"
            n54 = call "CaseTimer.vi"("CaseTime"=u32[] [2800, 2000, 1, 300, 1100, 1100, 876, 1] ("y"), "ElapsedTime"=w277) -> ("CaseNumber"=w278:i32)  [unwired: 9 in]
            "Waveform Chart 14" <- w278
            n55 = case shown="1" w278 {
              tunnel: w280 -> [w283 w289 w298]
              tunnel: [w282 w288 w294] -> w279
              frame 0 {
                # "Forward, Extend Arms"
                n56 = Bundle(cluster=w283, "X_axis"=0.0, "Y_axis"=-0.8, "RotationTarget"=0.0, "Arms"=0.8) -> (w282:T1)  [unwired: 3 in]
              }
              frame 1 {
                # "extend arms"
                n57 = Bundle(cluster=w289, "X_axis"=0.0, "Y_axis"=0.0, "RotationTarget"=0.0, "Arms"=0.8) -> (w288:T1)  [unwired: 3 in]
              }
              frame 2, Default {
                # "Stop"
                n58 = Bundle(cluster=w298, "X_axis"=0.0, "Y_axis"=0.0, "RotationTarget"=0.0, "Arms"=0.0) -> (w294:T1)  [unwired: 3 in]
              }
            }
          }
        }
      }
      frame "Auto_Switch_Postion_2" {
        n59 = case shown="\"L\", Default" w301 {
          tunnel: w300 -> [w307 w329]
          tunnel: [w306 w327] -> w299
          tunnel: w302 -> [w304 w331]
          frame "L", Default {
            # "Case:     Time:      Action:\n0               2000      Forward\n1"
            n60 = call "CaseTimer.vi"("CaseTime"=u32[] [2200, 750, 1, 500, 750, 600, 600, 2000, 1] ("y"), "ElapsedTime"=w304) -> ("CaseNumber"=w305:i32)  [unwired: 9 in]
            "Waveform Chart 42" <- w305
            n61 = case shown="1" w305 {
              tunnel: w307 -> [w310 w317 w326]
              tunnel: [w309 w316 w322] -> w306
              frame 0 {
                # "Forward  Extend Arms"
                n62 = Bundle(cluster=w310, "X_axis"=0.0, "Y_axis"=-0.8, "RotationTarget"=0.0, "Arms"=0.85) -> (w309:T1)  [unwired: 3 in]
              }
              frame 1 {
                # "Slide RIght Extend Arms"
                n63 = Bundle(cluster=w317, "X_axis"=0.0, "Y_axis"=0.0, "RotationTarget"=0.0, "ArmLift"=0.0, "Arms"=0.85) -> (w316:T1)  [unwired: 2 in]
              }
              frame 2, Default {
                # "Stop"
                n64 = Bundle(cluster=w326, "X_axis"=0.0, "Y_axis"=0.0, "RotationTarget"=0.0, "Arms"=0.0) -> (w322:T1)  [unwired: 3 in]
              }
            }
          }
          frame "R" {
            # "Case:     Time:     Action:\n0               2000     Forward, Extend Arms\n1                 750      Slide Right , Extend Arms\n2                 250      Forward, Extend Arms\n3               2000      Extend Arms, Release\n4                       1      Stop"
            n65 = call "CaseTimer.vi"("CaseTime"=u32[] [2000, 750, 700, 1, 1, 1000, 1000] ("y"), "ElapsedTime"=w331) -> ("CaseNumber"=w328:i32)  [unwired: 9 in]
            "Waveform Chart 43" <- w328
            n66 = case shown="2" w328 {
              tunnel: w329 -> [w334 w342 w348 w358]
              tunnel: [w333 w341 w347 w354] -> w327
              frame 0 {
                # "Forward, Extend Arms"
                n67 = Bundle(cluster=w334, "X_axis"=0.0, "Y_axis"=-0.8, "RotationTarget"=0.0, "Arms"=0.8) -> (w333:T1)  [unwired: 3 in]
              }
              frame 1 {
                # "Slide Right, Extend arms"
                n68 = Bundle(cluster=w342, "X_axis"=0.0, "Y_axis"=0.0, "RotationTarget"=0.0, "ArmLift"=0.0, "Hands"=0.0, "Arms"=0.85) -> (w341:T1)  [unwired: 1 in]
              }
              frame 2 {
                n69 = Bundle(cluster=w348, "X_axis"=0.0, "Y_axis"=0.0, "RotationTarget"=0.0, "ArmLift"=0.0, "Hands"=-0.6, "Arms"=0.85) -> (w347:T1)  [unwired: 1 in]
              }
              frame 3, Default {
                # "Stop"
                n70 = Bundle(cluster=w358, "X_axis"=0.0, "Y_axis"=0.0, "RotationTarget"=0.0) -> (w354:T1)  [unwired: 4 in]
              }
            }
          }
        }
      }
      frame "Auto_Switch_Postion_3" {
        n71 = case shown="\"R\", Default" w362 {
          tunnel: w361 -> [w367 w413]
          tunnel: [w366 w412] -> w360
          tunnel: w359 -> [w364 w410]
          frame "R", Default {
            # "Case:     Time:     Action:\n0               2800      Forward, Extend Arms\n1                 600      Rotate Left 90 deg, Extend Arms\n2                 400      Forward, Extend Arms\n3               1000      Extend Arms, Release Block\n4                       1       Stop"
            n72 = call "CaseTimer.vi"("CaseTime"=u32[] [2000, 660, 3000, 300, 1, 1000, 1000, 1] ("y"), "ElapsedTime"=w364) -> ("CaseNumber"=w365:i32)  [unwired: 9 in]
            "Waveform Chart 44" <- w365
            n73 = case shown="3" w365 {
              tunnel: w367 -> [w369 w375 w381 w391 w393 w399 w408]
              tunnel: [w368 w374 w380 w387 w392 w398 w404] -> w366
              frame 0 {
                # "Forward"
                n74 = Bundle(cluster=w369, "X_axis"=0.0, "Y_axis"=-1.0, "RotationTarget"=0.0) -> (w368:T1)  [unwired: 4 in]
              }
              frame 1 {
                # "Rotate Left 90 deg, Extend Arms"
                n75 = Bundle(cluster=w375, "X_axis"=-1.0, "Y_axis"=0.0, "RotationTarget"=0.0, "Arms"=0.8) -> (w374:T1)  [unwired: 3 in]
              }
              frame 2 {
                # "Forward, Extend Arms"
                n76 = Bundle(cluster=w381, "X_axis"=0.0, "Y_axis"=-1.0, "RotationTarget"=0.0, "Arms"=0.8) -> (w380:T1)  [unwired: 3 in]
              }
              frame 3 {
                # "Extend Arms, Release"
                n77 = Bundle(cluster=w391, "X_axis"=0.0, "Y_axis"=0.0, "RotationTarget"=0.0, "Hands"=-0.6, "Arms"=0.8) -> (w387:T1)  [unwired: 2 in]
              }
              frame 4 {
                # "backup"
                n78 = Bundle(cluster=w393, "X_axis"=0.0, "Y_axis"=1.0, "RotationTarget"=0.0, "Arms"=0.0) -> (w392:T1)  [unwired: 3 in]
              }
              frame 5 {
                # "slide left"
                n79 = Bundle(cluster=w399, "X_axis"=0.0, "Y_axis"=0.0, "RotationTarget"=0.7, "Arms"=0.0) -> (w398:T1)  [unwired: 3 in]
              }
              frame 6, Default {
                # "Stop"
                n80 = Bundle(cluster=w408, "X_axis"=0.0, "Y_axis"=0.0, "RotationTarget"=0.0) -> (w404:T1)  [unwired: 4 in]
              }
            }
          }
          frame "L" {
            # "Case:     Time:     Action:\n0               2800     Forward, Extend Arms\n1               2000      Extend Arms\n2                       1       Stop"
            n81 = call "CaseTimer.vi"("CaseTime"=u32[] [2500, 2000, 1, 1000, 1000, 1000, 1000] ("y"), "ElapsedTime"=w410) -> ("CaseNumber"=w411:i32)  [unwired: 9 in]
            "Waveform Chart 45" <- w411
            n82 = case shown="2, Default" w411 {
              tunnel: w413 -> [w416 w425 w431]
              tunnel: [w415 w421 w427] -> w412
              frame 0 {
                # "Drive Forward, Extend Arms"
                n83 = Bundle(cluster=w416, "X_axis"=0.0, "Y_axis"=-0.8, "RotationTarget"=0.0, "Arms"=0.8) -> (w415:T1)  [unwired: 3 in]
              }
              frame 1 {
                # "Extend Arms"
                n84 = Bundle(cluster=w425, "X_axis"=0.0, "Y_axis"=0.0, "RotationTarget"=0.0, "Arms"=0.8) -> (w421:T1)  [unwired: 3 in]
              }
              frame 2, Default {
                # "Stop"
                n85 = Bundle(cluster=w431, "X_axis"=0.0, "Y_axis"=0.0, "RotationTarget"=0.0, "Arms"=0.0) -> (w427:T1)  [unwired: 3 in]
              }
            }
          }
        }
      }
    }
    n86 = Unbundle By Name(w15) -> ("Lift"=w64:dbl)
    n87 = call "g_DI InputsALB.vi"("Action"=T2."read") -> ("DI out"=w55:T3)  [unwired: 10 in]
    n88 = Unbundle By Name(w14) -> ("X_axis"=w32:dbl, "Y_axis"=w31:dbl, "RotationTarget"=w30:dbl)
    "Waveform Chart 10" <- w30
    "Waveform Chart 15" <- w32
    "Waveform Chart 6" <- w31
    n89 = call "g_DI InputsALB.vi"("Action"=T2."read") -> ("DI out"=w61:T3)  [unwired: 10 in]
    n90 = call "g_DI InputsALB.vi"("Action"=T2."read") -> ("DI out"=w54:T3)  [unwired: 10 in]
    n91 = call "g_DI InputsALB.vi"("Action"=T2."read") -> ("DI out"=w37:T3)  [unwired: 10 in]
    n92 = Unbundle By Name(w18) -> ("Hands"=w19:dbl)
    n93 = Unbundle By Name(w16) -> ("ArmLift"=w41:dbl)
    n94 = Unbundle By Name(w61) -> ("DIO 0-LiftMinLimitSwitch"=w62:bool, "DIO 2-LiftArmMinLimitSwitch"=w63:bool)
    n95 = Unbundle By Name(w54) -> ("DIO 4-RightArmMaxLimitSwitch"=w47:bool, "DIO 5-RightArmMinLimitSwitch"=w46:bool)
    n96 = Unbundle By Name(w37) -> ("DIO 1-LiftMaxLimitSwitch"=w38:bool, "DIO 3-LiftArmMaxLimitSwitch"=w39:bool)
    n97 = Unbundle By Name(w55) -> ("DIO 6-LeftArmMaxLimitSwitch"=w45:bool, "DIO 7-LeftArmMinLimitSwitch"=w44:bool)
    n98 = Unbundle By Name(w17) -> ("Arms"=w56:dbl)
    n99 = call <vilib>:"WPI_MotorControlRefNum Registry Get.vi"("refnum name"="HandMotors") -> ("MotorControlDevRef"=w33:T4)  [unwired: 9 in, 1 out]
    n100 = call "DriveAutonomous.vi"("Rotation"=w30, "LY_Axis"=w31, "LX_Axis"=w32) -> ()  [unwired: 4 in, 5 out]
    n101 = call <vilib>:"WPI_MotorControlSetOutput.vi"("Output"=w19, "MotorControlDevRef"=w33) -> ()  [unwired: 7 in, 3 out]
    n102 = Not(x=w62) -> (.not. x?=w60:bool)
    "Lift Max Limit 2" <- w60
    n103 = Not(x=w38) -> (.not. x?=w35:bool)
    "Arm Lift Max Limit  2" <- w35
    n104 = Not(x=w45) -> (.not. x?=w52:bool)
    "Left Arm Max Limit 2" <- w52
    n105 = Not(x=w47) -> (.not. x?=w50:bool)
    "Right Arm Max Limit 2" <- w50
    n106 = Not(x=w63) -> (.not. x?=w59:bool)
    "Lift Min Limit  2" <- w59
    n107 = Not(x=w39) -> (.not. x?=w36:bool)
    "Arm Lift Min Limit  2" <- w36
    n108 = Not(x=w44) -> (.not. x?=w51:bool)
    "Left Arm Min Limit 2" <- w51
    n109 = Not(x=w46) -> (.not. x?=w49:bool)
    "Right Arm Min Limit 2" <- w49
    n110 = Multiply(x=w56, y=0.8) -> (x*y=w53:dbl)
    n111 = call "Motor Command with Limit Switches.vi"("LowLimitSwitch"=w59, "MotorCommandIn"=w64, "HighLimitSwitch"=w60) -> (0:w58:dbl)
    "LiftMotorCmd 2" <- w58
    n112 = call "Motor Command with Limit Switches.vi"("LowLimitSwitch"=w36, "MotorCommandIn"=w41, "HighLimitSwitch"=w35) -> (0:w40:dbl)
    "ArmLiftMotorCmd 2" <- w40
    n113 = call "Motor Command with Limit Switches.vi"("LowLimitSwitch"=w49, "MotorCommandIn"=w53, "HighLimitSwitch"=w50) -> (0:w13:dbl)
    "RightArmMotorCmd 2" <- w13
    n114 = call "Motor Command with Limit Switches.vi"("LowLimitSwitch"=w51, "MotorCommandIn"=w53, "HighLimitSwitch"=w52) -> (0:w48:dbl)
    "LeftArmMotorCmd 2" <- w48
    n115 = call <vilib>:"WPI_MotorControlRefNum Registry Get.vi"("refnum name"="LiftMotor") -> ("MotorControlDevRef"=w57:T4)  [unwired: 9 in, 1 out]
    n116 = call <vilib>:"WPI_MotorControlRefNum Registry Get.vi"("refnum name"="LeftArmMotor") -> ("MotorControlDevRef"=w43:T4)  [unwired: 9 in, 1 out]
    n117 = call <vilib>:"WPI_MotorControlRefNum Registry Get.vi"("refnum name"="ArmLiftMotor") -> ("MotorControlDevRef"=w34:T4)  [unwired: 9 in, 1 out]
    n118 = call <vilib>:"WPI_MotorControlRefNum Registry Get.vi"("refnum name"="RightArmMotor") -> ("MotorControlDevRef"=w42:T4)  [unwired: 9 in, 1 out]
    n119 = call <vilib>:"WPI_MotorControlSetOutput.vi"("Output"=w58, "MotorControlDevRef"=w57) -> ()  [unwired: 7 in, 3 out]
    n120 = call <vilib>:"WPI_MotorControlSetOutput.vi"("Output"=w48, "MotorControlDevRef"=w43) -> ()  [unwired: 7 in, 3 out]
    n121 = call <vilib>:"WPI_MotorControlSetOutput.vi"("Output"=w13, "MotorControlDevRef"=w42) -> ()  [unwired: 7 in, 3 out]
    n122 = call <vilib>:"WPI_MotorControlSetOutput.vi"("Output"=w40, "MotorControlDevRef"=w34) -> ()  [unwired: 7 in, 3 out]
    n123 = Wait (ms)(milliseconds to wait=u32 20) -> ()  [unwired: 1 out]
  }
